vi "curr.vi"() -> ()   [LabVIEW 2020]
panel:
  in  "stop (F)":bool
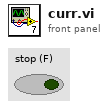
[diagram p1: front panel]
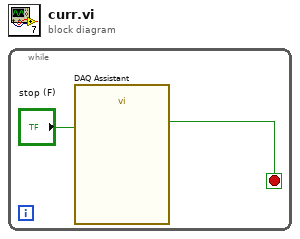
[diagram p0: block diagram]
diagram:
  n1 = while {
    stop <- w1 stop-if-true
    n2 = call "DAQ Assistant"("stop (F)"="stop (F)") -> ("stopped"=w1:bool)  [unwired: 15 in, 3 out]
  }
